vi "Close Audio File.vi"(8 "error in (no error)":errorcluster, 11 "Audio File Refnum In":refnum<file>) -> (0 "error out":errorcluster)   [LabVIEW 2020, in "G-Audio.lvlib"]
doc: "Close an audio file, and clean up the relevant decoder.\n\nThis node runs normally even if an error occurred before this node runs."
uses:
  G-Audio.lvlib
  <vilib>/Utility/error.llb/Error Cluster From Error Code.vi
  lib/g_audio_x86.dll
  lib/g_audio_x64.dll
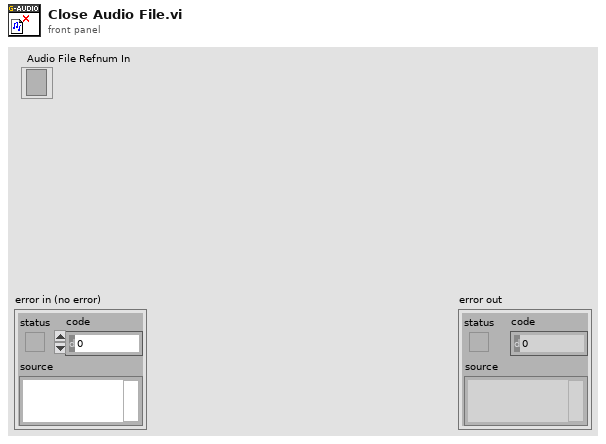
[diagram p1: front panel]
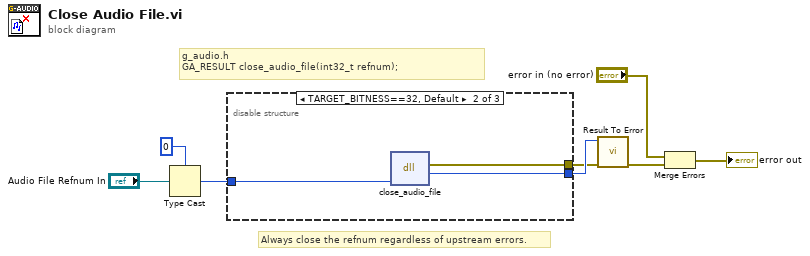
[diagram p0: block diagram]
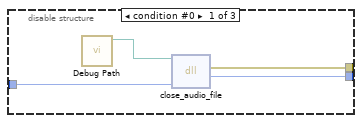
[diagram p2: hidden frame]
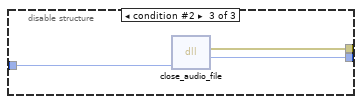
[diagram p3: hidden frame]
diagram:
  # "g_audio.h\nGA_RESULT close_audio_file(int32_t refnum);"
  # "Always close the refnum regardless of upstream errors."
  n1 = Type Cast(type=0, x="Audio File Refnum In") -> (*(type *) &x=w6:i32)
  n2 = disable-structure shown="TARGET_BITNESS==32, Default" {
    disable-tunnel: w6 -> [w12 w15 w18]
    disable-tunnel: [w11 w14 w17] -> w2
    disable-tunnel: [w10 w13 w16] -> w3
    frame condition #0 {
      n3 = call "Debug Path.vi"() -> ("Debug Path"=w9:path)  [unwired: 11 in]
      n4 = dll-call lib="?" fn="close_audio_file"(path in=w9, "refnum"=w12) -> (error out=w11:errorcluster, "result"=w10:i32)  [unwired: 3 in, 1 out]
    }
    frame condition #1 (active) {
      n5 = dll-call lib="C:/github/dataflowg/g-audio/src/LabVIEW/G-Audio/lib/g_audio_x86.*" fn="close_audio_file"("refnum"=w15) -> (error out=w14:errorcluster, "result"=w13:i32)  [unwired: 4 in, 1 out]
    }
    frame condition #2 {
      n6 = dll-call lib="C:/github/dataflowg/g-audio/src/LabVIEW/G-Audio/lib/g_audio_x64.*" fn="close_audio_file"("refnum"=w18) -> (error out=w17:errorcluster, "result"=w16:i32)  [unwired: 4 in, 1 out]
    }
  }
  n7 = call "Result To Error.vi"("error in (no error)"=w2, "Result Code"=w3) -> ("error out"=w1:errorcluster)  [unwired: 9 in]
  n8 = Merge Errors("error in (no error)", w1) -> (→"error out":errorcluster)
